vi "BuildTerminalLabelNameFromTerm.vi"(2 "Term":T1, 4 "VI Name":string) -> (0 "Label Name":string)   [LabVIEW 2012]
uses:
  <vilib>/XNodeSupport/XNodeTerm3.ctl
  <vilib>/XNodeSupport/XNodeString.ctl
  <vilib>/XNodeSupport/XNodeVariant.ctl
  <vilib>/XNodeSupport/XNodeRect32.ctl
  <vilib>/XNodeSupport/XNodeInt.ctl
  <vilib>/XNodeSupport/XNodeBool.ctl
  <vilib>/XNodeSupport/XNodeTermDirection.ctl
  CRef/CRef.lvlib
  <vilib>/XNodeSupport/NI_XNodeSupport.lvlib
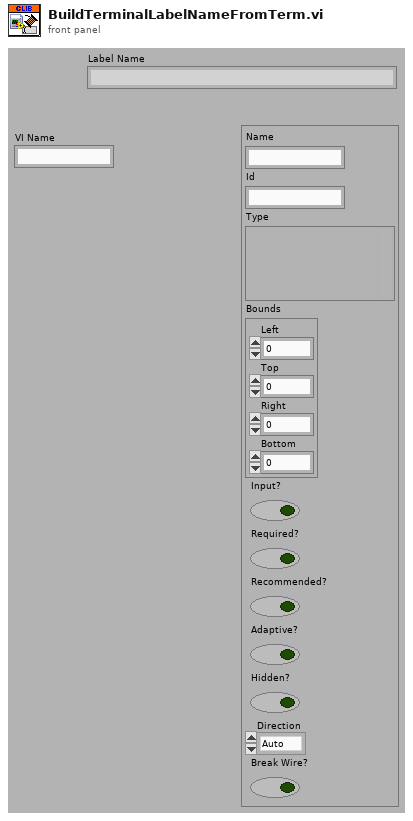
[diagram p1: front panel]
types:
  T1 = typedef "NI_XNodeSupport.lvlib/XNodeTerm3.ctl" = cluster{"Name":T2, "Id":T2, "Type":T3, "Bounds":T4, "Input?":T6, "Required?":T6, "Recommended?":T6, "Adaptive?":T6, "Hidden?":T6, "Direction":T7, "Break Wire?":T6}
  T2 = typedef "NI_XNodeSupport.lvlib/XNodeString.ctl" = string
  T3 = typedef "NI_XNodeSupport.lvlib/XNodeVariant.ctl" = variant
  T4 = typedef "NI_XNodeSupport.lvlib/XNodeRect32.ctl" = cluster{"Left":T5, "Top":T5, "Right":T5, "Bottom":T5}
  T5 = typedef "NI_XNodeSupport.lvlib/XNodeInt.ctl" = i32
  T6 = typedef "NI_XNodeSupport.lvlib/XNodeBool.ctl" = bool
  T7 = typedef "NI_XNodeSupport.lvlib/XNodeTermDirection.ctl" = enum32{"Auto", "Up", "Down", "Left", "Right", "Center"}
  T8 = typedef "CRef.lvlib/Master Types.ctl" = enum8{"Null", "Boolean", "U8", "I8", "U16", "I16", "U32", "I32", "U64", "I64", "Single", "Double", "Extended", "CSG", "CDB", "CXT", "Boolean(Def)", "U8(Def)", "I8(Def)", "U16(Def)", "I16(Def)", "U32(Def)", "I32(Def)", "Reserved Def", "Reserved Def1", "Single(Def)", "Double(Def)", "Reserved Def2", "Reserved Def3", "Reserved Def4", "Reserved Def5", "Unsigned(Def)", "Signed(Def)", "Real(Def)", "Reserved Def6", "Numeric(Def)", "String"}
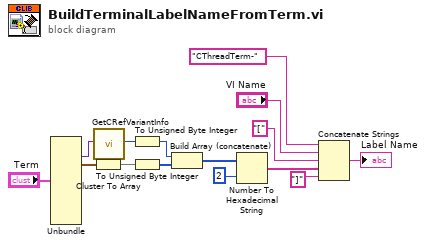
[diagram p0: block diagram]
diagram:
  n1 = Unbundle("Term") -> ("Type"=w1:T3, "Bounds"=w3:T4)  [unwired: 9 out]
  n2 = Cluster To Array(cluster=w3) -> (array=w14:T5[])
  n3 = call "GetCRefVariantInfo.vi"("variant"=w1) -> ("CRef Type"=w2:T8)  [unwired: 18 in]
  n4 = To Unsigned Byte Integer(number=w2) -> (unsigned 8bit integer=w12:u8)
  n5 = To Unsigned Byte Integer(number=w14) -> (unsigned 8bit integer=w13:u8[])
  n6 = Build Array (concatenate)(w12, w13) -> (w8:u8[])
  n7 = Number To Hexadecimal String(1:i16 2 ("width (-)"), 2:w8) -> (0:w7:string[])
  n8 = Concatenate Strings("CThreadTerm-", "VI Name", "[" ("string"), w7, "]" ("string")) -> (→"Label Name":string)
